vi "Sort.vi"() -> ()   [LabVIEW 2018]
panel:
  out "sorted array":string[](array[string])
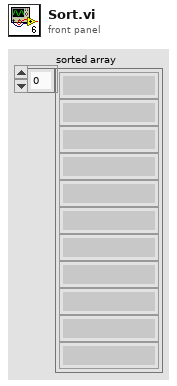
[diagram p1: front panel]
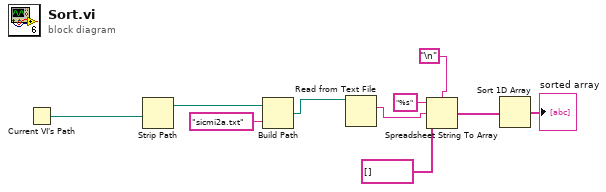
[diagram p0: block diagram]
diagram:
  n1 = Current VI's Path() -> (path=w8:path)
  n2 = Strip Path(path=w8) -> (stripped path=w10:path)  [unwired: 1 out]
  n3 = Build Path(base path=w10, name or relative path="sicmi2a.txt") -> (appended path=w7:path)
  n4 = Read from Text File(file (use dialog)=w7) -> (text=w5:string)  [unwired: 3 in, 3 out]
  n5 = Spreadsheet String To Array(delimiter (Tab)="\n", format string="%s", spreadsheet string=w5, array type (2D Dbl)=string[] []) -> (array=w2:string[])
  n6 = Sort 1D Array(array=w2) -> (sorted array=→"sorted array":string[])
